vi "Write.vi"(8 "Error In":errorcluster, 11 "SerialComm in":refnum<class "SerialComm.lvclass">) -> (0 "Error Out":errorcluster, 3 "SerialComm out":refnum<class "SerialComm.lvclass">)   [LabVIEW 2017, in "SerialComm.lvclass"]
uses:
  SerialComm.lvclass
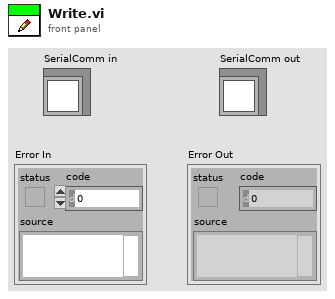
[diagram p1: front panel]
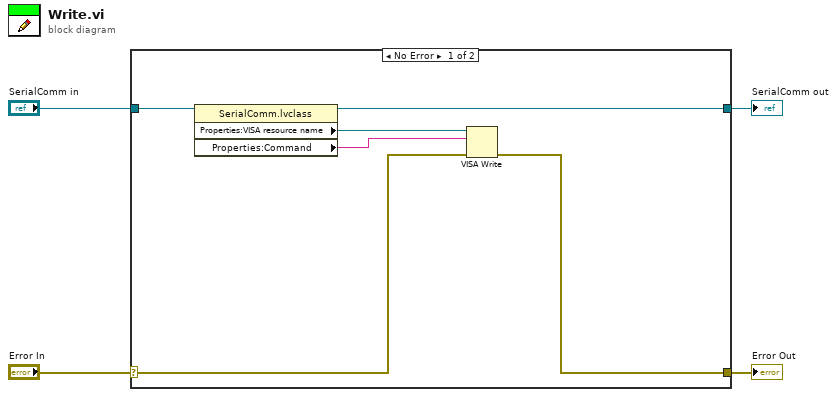
[diagram p0: block diagram]
diagram:
  n1 = case shown="No Error" "Error In" {
    selector: "Error In" -> [w6 w12]
    tunnel: [w5 w12] -> w3
    tunnel: [w9 w11] -> w1
    tunnel: "SerialComm in" -> [w10 w11]
    frame No Error {
      n2 = property class="SerialComm.lvclass"(reference=w10) -> (reference out=w9:refnum<class "SerialComm.lvclass">, "Properties:VISA resource name"=w8:refnum<visa-resource-name>, "Properties:Command"=w7:string)  [unwired: 1 in, 1 out]
      n3 = VISA Write(VISA resource name=w8, write buffer=w7, error in (no error)=w6) -> (error out=w5:errorcluster)  [unwired: 2 out]
    }
    frame Error {
    }
  }
  "Error Out" <- w3
  "SerialComm out" <- w1
